vi "SCXI-1125 Temperature Reader.vi"() -> ()   [LabVIEW 2010]
panel:
  in  "rate":dbl=60.0 format="%0.2f"
  in  "samples per channel":i32=100
  in  "stop":bool
  out "Limit Exceeded?":bool
  in  "DAQmx Channel Name":refnum<k21>
  in  "Temperature Limit":dbl(slide) scale=20.0..40.0
  out "Temperature Chart":cluster{"Temperature Limit":dbl, "data":dbl}(graph)
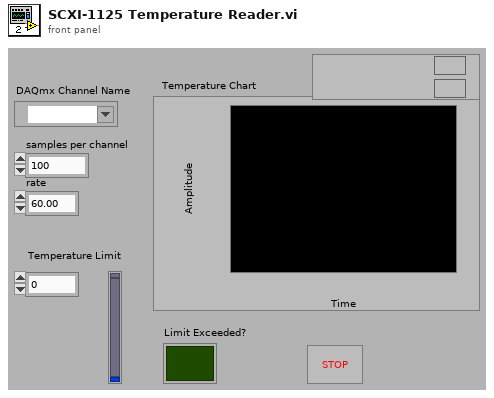
[diagram p1: front panel]
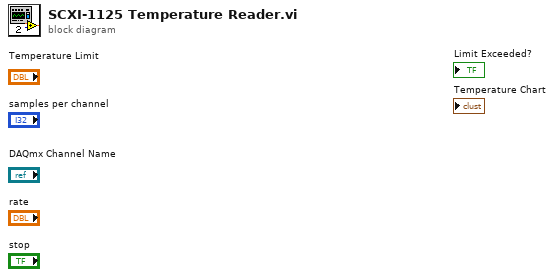
[diagram p0: block diagram]
diagram:
